vi "41_base_image.vi"() -> ()   [LabVIEW 2018]
panel:
  in  "Stop (F)":bool
  out "Image Out":T1(plugin-control)
  # "ъ瓜"
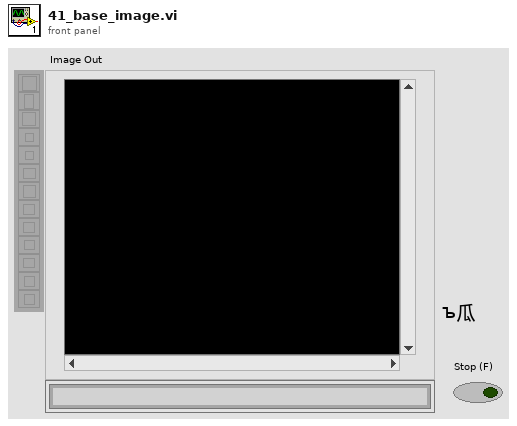
[diagram p1: front panel]
types:
  T1 = typedef "IMAQ Image.ctl" = refnum<image>
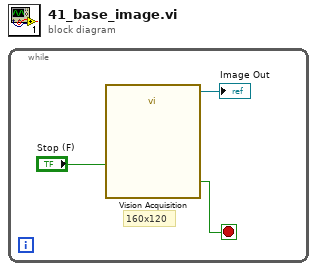
[diagram p0: block diagram]
diagram:
  n1 = while {
    stop <- w2 stop-if-true
    # "160x120"
    n2 = call "Vision Acquisition"("Stop (F)"="Stop (F)") -> ("Image Out"=→"Image Out":T1, "Stopped"=w2:bool)  [unwired: 24 in, 1 out]
  }
